vi "Y stage safety.vi"(7 "new position":dbl format="%#_13g", 8 "Error In":errorcluster, 10 "Table Stages":T1={"X Stage"={"Position"=0.0, "Is.Enabled?"=FALSE, "Is.Connected?"=FALSE, "Device SN"="45876539", "AccelerationMaximum"=0.0, "VelocityMaximum"=0.0, "Acceleration"=0.0, "Velocity"=0.0, "waitTimeout (ms)"=0, "Model"=enum."None", "Is.Homed?"=FALSE, "MOVE"=FALSE}, "Y Stage"={"Position"=0.0, "Is.Enabled?"=FALSE, "Is.Connected?"=FALSE, "Device SN"="45876539", "AccelerationMaximum"=0.0, "VelocityMaximum"=0.0, "Acceleration"=0.0, "Velocity"=0.0, "waitTimeout (ms)"=0, "Model"=enum."None", "Is.Homed?"=FALSE, "MOVE"=FALSE}, "Z Stage"={"Position"=0.0, "Is.Enabled?"=FALSE, "Is.Connected?"=FALSE, "Device SN"="45876539", "AccelerationMaximum"=0.0, "VelocityMaximum"=0.0, "Acceleration"=0.0, "Velocity"=0.0, "waitTimeout (ms)"=0, "Model"=enum."None", "Is.Homed?"=FALSE, "MOVE"=FALSE}, "Attenuator"={"Position"=0.0, "Is.Enabled?"=FALSE, "Is.Connected?"=FALSE, "Device SN"="45876539", "AccelerationMaximum"=0.0, "VelocityMaximum"=0.0, "Acceleration"=0.0, "Velocity"=0.0, "waitTimeout (ms)"=0, "Model"=enum."None", "Is.Homed?"=FALSE, "MOVE"=FALSE}}) -> (0 "Error Out":errorcluster, 1 "crash?":bool)   [LabVIEW 2018]
uses:
  Controls/Translation Stage Parameters.ctl
  Hardware Mfg/Thorlabs Translation Stages/Controls/Translation Stage Cluster.ctl
  Controls/Translation Stage Types.ctl
  Controls/Set Get Controls.ctl
  Hardware Mfg/Thorlabs Translation Stages/Controls/Motion Translation Module Control2.ctl
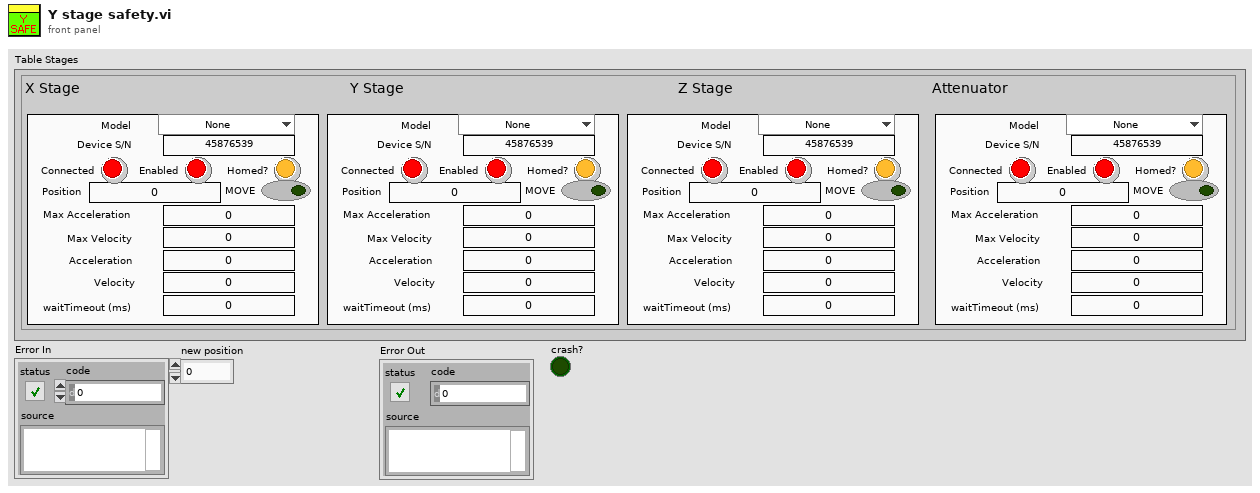
[diagram p1: front panel]
types:
  T1 = typedef "Translation Stage Parameters.ctl" = cluster{"X Stage":T2, "Y Stage":T2, "Z Stage":T2, "Attenuator":T2}
  T2 = typedef "Translation Stage Cluster.ctl" = cluster{"Position":dbl, "Is.Enabled?":bool, "Is.Connected?":bool, "Device SN":string, "AccelerationMaximum":dbl, "VelocityMaximum":dbl, "Acceleration":dbl, "Velocity":dbl, "waitTimeout (ms)":i32, "Model":T3, "Is.Homed?":bool, "MOVE":bool}
  T3 = typedef "Translation Stage Types.ctl" = enum16{"None", "Thorlabs LTS", "Thorlabs MLJ"}
  T4 = typedef "Motion Translation Module Control2.ctl" = enum16{"Init", "Home", "Status", "Velocity/Accel", "Position", "Jog", "Stop", "Uninit", "Enable", "Disable"}
  T5 = typedef "Set Get Controls.ctl" = enum16{"Set", "Get"}
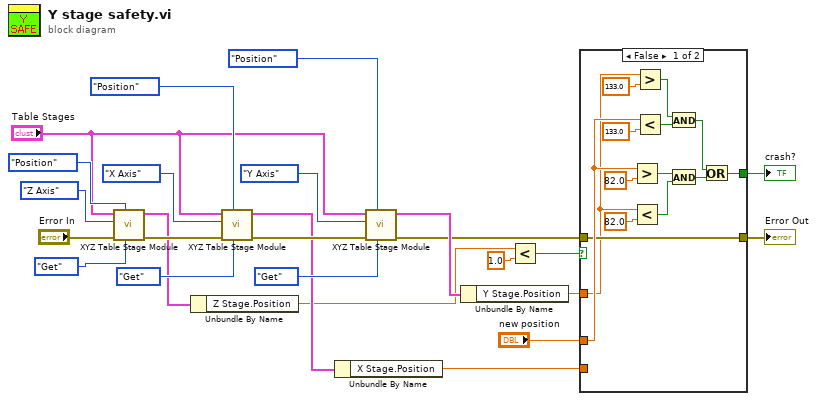
[diagram p0: block diagram]
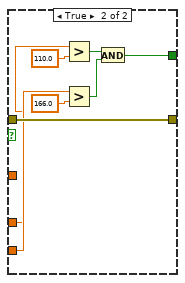
[diagram p2: hidden frame]
diagram:
  n1 = call "XYZ Table Stage Module.vi"("Set/Get"=Set_Get_Controls."Get", "Action"=Motion_Translation_Module_Control2."Position", "Error In"="Error In", "Axis"=enum16{"X Axis", "Y Axis", "Z Axis"}."Z Axis", "Table Stages"="Table Stages") -> ("Error Out"=w18:errorcluster, "Table Stages [out]"=w13:T1)  [unwired: 5 in]
  n2 = Unbundle By Name(w13) -> ("Z Stage.Position"=w10:dbl)
  n3 = call "XYZ Table Stage Module.vi"("Set/Get"=Set_Get_Controls."Get", "Action"=Motion_Translation_Module_Control2."Position", "Error In"=w18, "Axis"=enum16{"X Axis", "Y Axis", "Z Axis"}."X Axis", "Table Stages"="Table Stages") -> ("Error Out"=w14:errorcluster, "Table Stages [out]"=w11:T1)  [unwired: 5 in]
  n4 = Unbundle By Name(w11) -> ("X Stage.Position"=w4:dbl)
  n5 = call "XYZ Table Stage Module.vi"("Set/Get"=Set_Get_Controls."Get", "Action"=Motion_Translation_Module_Control2."Position", "Error In"=w14, "Axis"=enum16{"X Axis", "Y Axis", "Z Axis"}."Y Axis", "Table Stages"="Table Stages") -> ("Error Out"=w2:errorcluster, "Table Stages [out]"=w12:T1)  [unwired: 5 in]
  n6 = Unbundle By Name(w12) -> ("Y Stage.Position"=w6:dbl)
  n7 = Less?(x=w10, y=1.0) -> (x < y?=w8:bool)
  n8 = case shown="False" w8 {
    tunnel: "new position" -> [w33 w40]
    tunnel: w6 -> [w26 _]
    tunnel: [w28 w43] -> w5
    tunnel: w4 -> [_ w41]
    tunnel: w2 -> [w27 w42]
    tunnel: [w27 w42] -> w1
    frame False {
      n9 = Greater?(x=w33, y=82.0) -> (0:w32:bool)
      n10 = Less?(x=w26, y=82.0) -> (x < y?=w31:bool)
      n11 = Greater?(x=w26, y=133.0) -> (0:w37:bool)
      n12 = Less?(x=w33, y=133.0) -> (x < y?=w36:bool)
      n13 = And(x=w37, y=w36) -> (x .and. y?=w30:bool)
      n14 = And(x=w32, y=w31) -> (x .and. y?=w29:bool)
      n15 = Or(x=w30, y=w29) -> (x .or. y?=w28:bool)
    }
    frame True {
      n16 = Greater?(x=w40, y=110.0) -> (0:w45:bool)
      n17 = Greater?(x=w41, y=166.0) -> (0:w44:bool)
      n18 = And(x=w45, y=w44) -> (x .and. y?=w43:bool)
    }
  }
  "crash?" <- w5
  "Error Out" <- w1
